vi "Receive Dashboard Packet.vi"(7 "connection ID":refnum<k16>) -> ()   [LabVIEW 2014]
uses:
  Common Code/Dashboard Control Data.ctl
  Common Code/Roller Control.ctl
  Common Code/Elevator DB Control.ctl
  Common Code/Elevator Presets.ctl
  Common Code/Encoder Control.ctl
  Common Code/Drivetrain Settings.ctl
  Pike/Pike DB Controls.ctl
  Robot Global Data.vi
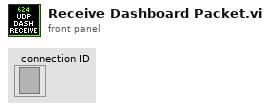
[diagram p1: front panel]
types:
  T1 = typedef "Dashboard Control Data.ctl" = cluster{"Cam Exposure":dbl, "Go to angle":dbl, "Steer PID Gains":cluster{"proportional gain (Kc)":dbl, "integral time (Ti, min)":dbl, "derivative time (Td, min)":dbl}, "Steer PID output Range":cluster{"output high":dbl, "output low":dbl}, "Pressure m \nValue":dbl, "Pressure b \nValue":dbl, "Roller Command Cluster ":T2, "Elevator":T3, "Encoder Control":T5, "Auton Settings":cluster{"Drive Dist Window Size":dbl}, "Drivetrain Settings":T6, "Lance":T7}
  T2 = typedef "Roller Control.ctl" = cluster{"Intake Speed":dbl, "Turn In Speed":dbl, "Unload Speed":dbl, "Turn Out Speed":dbl, "Ping Align Tolerance":dbl, "Tote Range Threshold":dbl, "Right Pot 0":dbl, "Pot Threshold":dbl, "Left Pot 0":dbl, "Right Pot Scale":dbl, "Left Pot Scale":dbl, "Min Elevator Height":dbl, "Eject Time":dbl, "Eject US Threshold":dbl, "Anti-Twitch Time":u32, "Ping Caring Threshold":dbl, "Pot Diff Threshold":dbl, "Pinch Sustain":u32, "Absorb Give Up Threshold":dbl, "Untip In Threshold":dbl, "Untip Grab Range":dbl, "Ultrasonic Hold Time":u32, "Landscape Absorb Time":u32, "Pot Use Wait Time":u32, "Can Turn Stop Range":dbl, "HP Load Speed":dbl}
  T3 = typedef "Elevator DB Control.ctl" = cluster{"PID Output Range":cluster{"output high":dbl, "output low":dbl}, "PID gains":cluster{"proportional gain (Kc)":dbl, "integral time (Ti, min)":dbl, "derivative time (Td, min)":dbl}, "Height Tolerance":sgl, " Encoder Constant":dbl, "Eject Time":sgl, "Zeroing Speed":sgl, "Presets":T4, "Ping Detect Threshold":sgl, "Trashcan Detect Threshold":sgl, "Zero Filter Time":dbl, "Stabilizer Open Time":dbl, "Zero Creep Speed":dbl, "Max Current":dbl, "Current Trip Time":dbl, "Abort Pitch":dbl, "Finger m":dbl, "Finger b":dbl, "Finger max ":dbl, "Finger Stabilizer":dbl, "Finger Store":dbl, "Finger Stop Store":dbl, "Stabilizer Close Time":dbl, "Finger min":dbl, "Unstick gain":dbl}
  T4 = typedef "Elevator Presets.ctl" = cluster{"Pickup 2 w/ Tote":sgl, "Pickup 2 w/ Trashcan":sgl, "Pickup 3 w/ Tote":sgl, "Pickup 3 w/ Trashcan":sgl, "Bottom":sgl, "Pickup 1 w/ Tote":sgl, "Pickup Trashcan":sgl, "Pickup 1 w/ Trashcan":sgl, "Eject":sgl, "Hold Low":sgl, "Step add height":sgl, "Untip Lift":dbl, "Drop Stack":dbl, "HP Load Hold":dbl, "HP Load Drop":dbl, "HP Load Hold Can":dbl, "Store can max":dbl, "HP Drag Score":dbl, "HP Drag Finish":dbl, "Finger trashcan avoid":dbl}
  T5 = typedef "Encoder Control.ctl" = cluster{"Left Tick Constant":dbl, "Right Tick Constant":dbl, "Center Tick Constant":dbl, "Reset?":bool, "Y Dist":cluster{"PID gains":cluster{"proportional gain (Kc)":dbl, "integral time (Ti, min)":dbl, "derivative time (Td, min)":dbl}}, "X Dist":cluster{"PID gains":cluster{"proportional gain (Kc)":dbl, "integral time (Ti, min)":dbl, "derivative time (Td, min)":dbl}}, "Y Stop Thresh":dbl, "Y Stop Speed":dbl, "X Stop Thresh":dbl, "X Stop Speed":dbl}
  T6 = typedef "Drivetrain Settings.ctl" = cluster{"Gyro Tolerance":sgl, "Strafe Correct max steer":sgl, "Strafe Timer Wait":sgl, "Throttle Ramp (ms)":sgl, "Strafe Ramp (ms)":sgl, "Angular rate compensation":bool, "Throttle to Rate Scale":sgl, "Rate compensation gain":sgl, "Creep Steer":sgl, "Creep Throttle":sgl}
  T7 = typedef "Pike DB Controls.ctl" = cluster{"Down Speed":dbl, "Up Speed":dbl, "Max Down Time":dbl, "Max Up Time":dbl, "Current Limit":dbl}
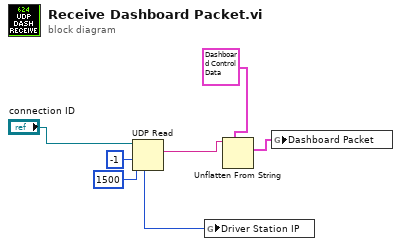
[diagram p0: block diagram]
diagram:
  n1 = UDP Read(connection ID="connection ID", max size (548)=1500, timeout ms (25000)=-1) -> (data out=w7:string, 6:w4:u32)  [unwired: 1 in, 3 out]
  n2 = global write "Robot Global Data.vi" "Driver Station IP"(w4) -> ()
  n3 = Unflatten From String(type=T1 {"Cam Exposure"=0.0, "Go to angle"=0.0, "Steer PID Gains"={"proportional gain (Kc)"=1.0, "integral time (Ti, min)"=0.01, "derivative time (Td, min)"=0.0}, "Steer PID output Range"={"output high"=1.0, "output low"=-1.0}, "Pressure m \nValue"=0.0, "Pressure b \nValue"=0.0, "Roller Command Cluster "={"Intake Speed"=0.0, "Turn In Speed"=0.0, "Unload Speed"=0.0, "Turn Out Speed"=0.0, "Ping Align Tolerance"=0.0, "Tote Range Threshold"=0.0, "Right Pot 0"=0.0, "Pot Threshold"=0.0, "Left Pot 0"=0.0, "Right Pot Scale"=0.0, "Left Pot Scale"=0.0, "Min Elevator Height"=0.0, "Eject Time"=0.0, "Eject US Threshold"=0.0, "Anti-Twitch Time"=0, "Ping Caring Threshold"=0.0, "Pot Diff Threshold"=0.0, "Pinch Sustain"=0, "Absorb Give Up Threshold"=0.0, "Untip In Threshold"=0.0, "Untip Grab Range"=0.0, "Ultrasonic Hold Time"=0, "Landscape Absorb Time"=0, "Pot Use Wait Time"=0, "Can Turn Stop Range"=0.0, "HP Load Speed"=0.0}, "Elevator"={"PID Output Range"={"output high"=100.0, "output low"=-100.0}, "PID gains"={"proportional gain (Kc)"=1.0, "integral time (Ti, min)"=0.01, "derivative time (Td, min)"=0.0}, "Height Tolerance"=0.0, " Encoder Constant"=0.0, "Eject Time"=0.0, "Zeroing Speed"=0.0, "Presets"={"Pickup 2 w/ Tote"=0.0, "Pickup 2 w/ Trashcan"=0.0, "Pickup 3 w/ Tote"=0.0, "Pickup 3 w/ Trashcan"=0.0, "Bottom"=0.0, "Pickup 1 w/ Tote"=0.0, "Pickup Trashcan"=0.0, "Pickup 1 w/ Trashcan"=0.0, "Eject"=0.0, "Hold Low"=0.0, "Step add height"=0.0, "Untip Lift"=0.0, "Drop Stack"=0.0, "HP Load Hold"=0.0, "HP Load Drop"=0.0, "HP Load Hold Can"=0.0, "Store can max"=0.0, "HP Drag Score"=0.0, "HP Drag Finish"=0.0, "Finger trashcan avoid"=0.0}, "Ping Detect Threshold"=0.0, "Trashcan Detect Threshold"=0.0, "Zero Filter Time"=0.0, "Stabilizer Open Time"=0.0, "Zero Creep Speed"=0.0, "Max Current"=0.0, "Current Trip Time"=0.0, "Abort Pitch"=0.0, "Finger m"=0.0, "Finger b"=0.0, "Finger max "=0.0, "Finger Stabilizer"=0.0, "Finger Store"=0.0, "Finger Stop Store"=0.0, "Stabilizer Close Time"=0.0, "Finger min"=0.0, "Unstick gain"=0.0}, "Encoder Control"={"Left Tick Constant"=1.0, "Right Tick Constant"=0.0, "Center Tick Constant"=0.0, "Reset?"=FALSE, "Y Dist"={"PID gains"={"proportional gain (Kc)"=1.0, "integral time (Ti, min)"=0.0, "derivative time (Td, min)"=0.0}}, "X Dist"={"PID gains"={"proportional gain (Kc)"=1.0, "integral time (Ti, min)"=0.0, "derivative time (Td, min)"=0.0}}, "Y Stop Thresh"=0.0, "Y Stop Speed"=0.0, "X Stop Thresh"=0.0, "X Stop Speed"=0.0}, "Auton Settings"={"Drive Dist Window Size"=0.0}, "Drivetrain Settings"={"Gyro Tolerance"=0.0, "Strafe Correct max steer"=0.4, "Strafe Timer Wait"=250.0, "Throttle Ramp (ms)"=0.0, "Strafe Ramp (ms)"=0.0, "Angular rate compensation"=FALSE, "Throttle to Rate Scale"=0.0, "Rate compensation gain"=0.0, "Creep Steer"=0.0, "Creep Throttle"=0.0}, "Lance"={"Down Speed"=0.0, "Up Speed"=0.0, "Max Down Time"=0.0, "Max Up Time"=0.0, "Current Limit"=0.0}} ("DB Control Data"), binary string=w7) -> (value=w5:T1)  [unwired: 3 in, 2 out]
  n4 = global write "Robot Global Data.vi" "Dashboard Packet"(w5) -> ()
